vi "Connect.vi"(6 "Timeout (ms)":i32=5000, 8 "error in (no error)":errorcluster, 9 "Port":i32=851, 10 "Net ID":string) -> (0 "error out":errorcluster, 3 "TwinCAT ADS out":refnum<class "TwinCAT ADS.lvclass">)   [LabVIEW 2018, in "TwinCAT ADS.lvclass"]
uses:
  TwinCAT ADS.lvclass
  TwinCAT.Ads
  TwinCAT ADS.lvclass/TwinCAT ADS.ctl
panel:
  in  "TwinCAT ADS in":refnum<class "TwinCAT ADS.lvclass">
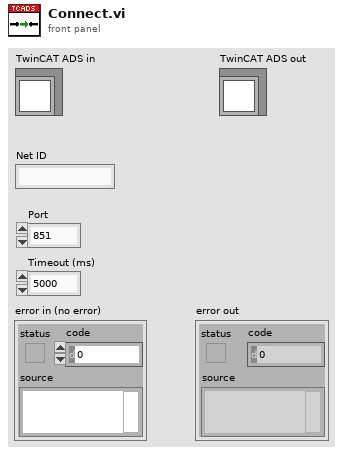
[diagram p1: front panel]
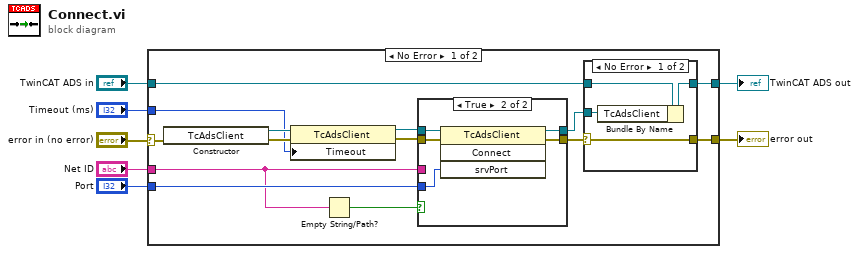
[diagram p0: block diagram]
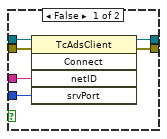
[diagram p3: hidden frame]
diagram:
  n1 = case shown="No Error" "error in (no error)" {
    selector: "error in (no error)" -> [w20 w40]
    tunnel: [w9 w40] -> w6
    tunnel: [w11 w39] -> w4
    tunnel: "TwinCAT ADS in" -> [w12 w39]
    tunnel: "Net ID" -> [w19 _]
    tunnel: "Port" -> [w21 _]
    tunnel: "Timeout (ms)" -> [w8 _]
    frame No Error {
      n2 = constructor class="TcAdsClient"(error in=w20) -> (reference out=w16:refnum<k24>, error out=w17:errorcluster)  [unwired: 2 in, 1 out]
      n3 = property class="TcAdsClient"(reference=w16, error in=w17, "Timeout"=w8) -> (reference out=w14:refnum<k24>, error out=w15:errorcluster)
      n4 = Empty String/Path?(string/path=w19) -> (empty?=w18:bool)
      n5 = case shown="True" w18 {
        tunnel: w15 -> [w33 w38]
        tunnel: w21 -> [w32 w35]
        tunnel: w14 -> [w31 w37]
        tunnel: [w30 w36] -> w13
        tunnel: w19 -> [w29 _]
        tunnel: [w28 w34] -> w10
        frame False {
          n6 = invoke class="TcAdsClient" method="Connect"(reference=w31, error in=w33, "netID"=w29, "srvPort"=w32) -> (reference out=w28:refnum<k24>, error out=w30:errorcluster)  [unwired: 1 in, 3 out]
        }
        frame True {
          n7 = invoke class="TcAdsClient" method="Connect"(reference=w37, error in=w38, "srvPort"=w35) -> (reference out=w34:refnum<k24>, error out=w36:errorcluster)  [unwired: 1 in, 2 out]
        }
      }
      n8 = case shown="No Error" w13 {
        selector: w13 -> [w22 w26]
        tunnel: w12 -> [w25 w27]
        tunnel: [w24 w27] -> w11
        tunnel: w10 -> [w23 _]
        tunnel: [w22 w26] -> w9
        frame No Error {
          n9 = Bundle By Name(cluster=w25, "TcAdsClient"=w23) -> (w24:refnum<class "TwinCAT ADS.lvclass">)
        }
        frame Error {
        }
      }
    }
    frame Error {
    }
  }
  "error out" <- w6
  "TwinCAT ADS out" <- w4
